vi "DragDropCustomize.vi"(5 "Set Cursor (T)":bool=TRUE, 7 "Function":enum16{"Event", "Cleanup"}(ring), 8 "error in (no error)":errorcluster, 9 "Coords":T2, 10 "CtlRef":refnum<vi>, 11 "Event Type":T3) -> (0 "error out":errorcluster, 1 "InBounds":bool, 2 "CtlRef out":refnum<vi>, 3 "Drag Status":T1, 4 "Bar Cursor ID":refnum<k1>)   [LabVIEW 2021, in "TreeControlLib.lvlib"]
uses:
  TreeControlLib.lvlib
  <vilib>/event_ctls.llb/lveventtype.ctl
  <vilib>/Utility/miscctls.llb/LVPoint32TypeDef.ctl
  ce4e9e53-98d0-488d-9291-147195c1407e.vi
  <vilib>/Utility/cursorutil.llb/Set Cursor (Icon Pict).vi
  <vilib>/Utility/cursorutil.llb/Set Cursor (Cursor ID).vi
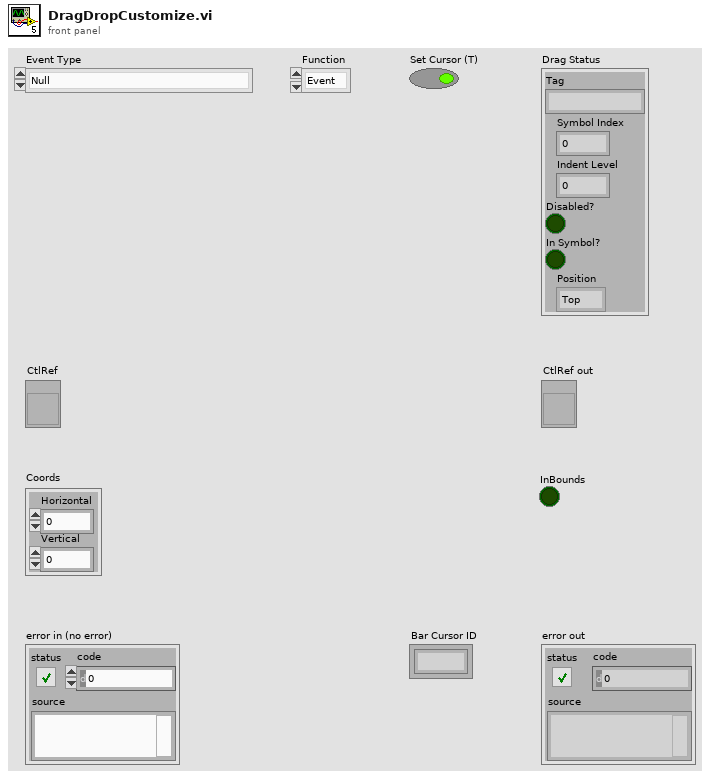
[diagram p1: front panel]
types:
  T1 = cluster{"Tag":string, "Symbol Index":i32, "Indent Level":i32, "Disabled?":bool, "In Symbol?":bool, "Position":enum16{"Top", "Center", "Bottom"}}
  T2 = typedef "LVPoint32TypeDef.ctl" = cluster{"Horizontal":i32, "Vertical":i32}
  T3 = typedef "lveventtype.ctl" = enum32{"Null", "Timeout", "Annotation Menu Selection", "Annotation Menu Selection?", "App Instance Close", "App Instance Close?", "Autoscale Range Change", "Bookmark Info Change", "Cell Edit", "Cell Edit?", "Cursor Grab", "Cursor Grab?", "Cursor Menu Selection", "Cursor Menu Selection?", "Cursor Move", "Cursor Release", "Data Change", "Direction Change", "Display State Change", "Drag Ended", "Drag Enter", "Drag Leave", "Drag Over", "Drag Source Update", "Drag Starting", "Drag Starting?", "Drop", "Exec State Change", "Key Down", "Key Down?", "Key Repeat", "Key Repeat?", "Key Up", "Listbox Double Click", "Menu Activation?", "Menu Selection (App)", "Menu Selection? (App)", "Menu Selection (User)", "Mouse Down", "Mouse Down?", "Mouse Enter", "Mouse Leave", "Mouse Move", "Mouse Up", "Mouse Wheel", "NI Security User Change (App)", "Pane Size", "Panel Close", "Panel Close?", "Panel Resize", "Plot Attribute Change", "Scale Range Change", "Shortcut Menu Activation?", "Shortcut Menu Selection (App)", "Shortcut Menu Selection? (App)", "Shortcut Menu Selection (User)", "Tree Double Click", "Tree Drag", "Tree Drag?", "Tree Drop", "Tree Drop?", "Tree Item Close", "Tree Item Close?", "Tree Item Open", "Tree Item Open?", "User Event", "Value Change"}
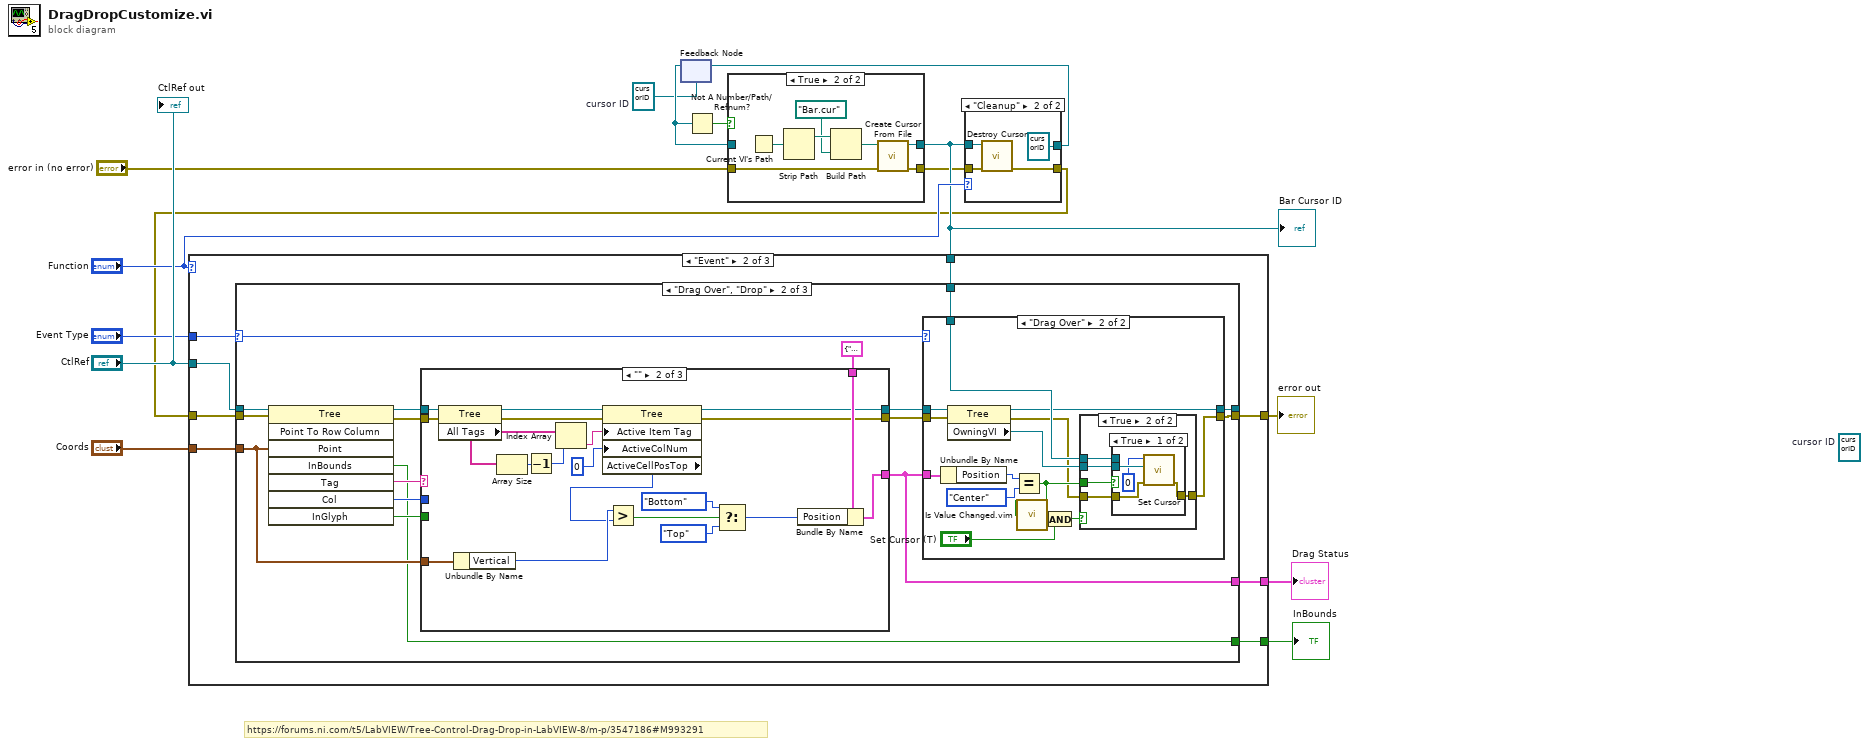
[diagram p0: block diagram]
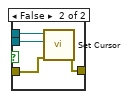
[diagram p6: hidden frame]
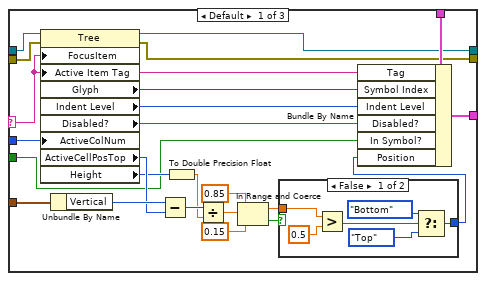
[diagram p7: hidden frame]
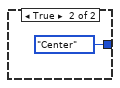
[diagram p8: hidden frame]
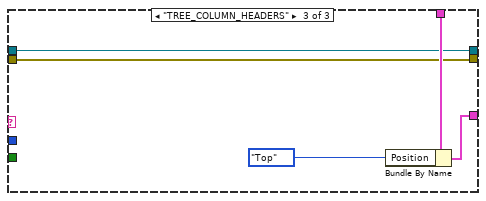
[diagram p9: hidden frame]
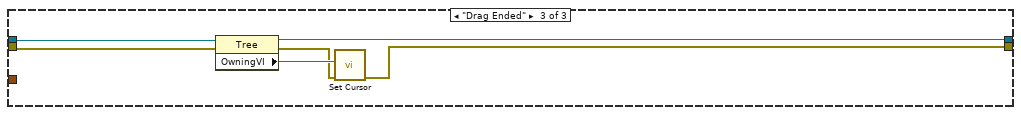
[diagram p10: hidden frame]
diagram:
  w2 = refnum<k1> refnum  # cursor ID
  (unwired) refnum<k1> refnum  # cursor ID
  # "https://forums.ni.com/t5/LabVIEW/Tree-Control-Drag-Drop-in-LabVIEW-8/m-p/3547186#M993291"
  n1 = feedback #1(w2) -> (w14:refnum<k1>)
  n2 = Not A Number/Path/Refnum?(number/path/refnum=w14) -> (NaN/Path/Refnum?=w15:bool)
  n3 = case shown="True" w15 {
    tunnel: w14 -> [w17 _]
    tunnel: [w17 w21] -> w8
    tunnel: "error in (no error)" -> [w16 w20]
    tunnel: [w16 w19] -> w4
    frame False {
    }
    frame True {
      n4 = Current VI's Path() -> (path=w24:path)
      n5 = Strip Path(path=w24) -> (stripped path=w22:path)  [unwired: 1 out]
      n6 = Build Path(base path=w22, name or relative path=path "Bar.cur" ("cursor file")) -> (appended path=w23:path)
      n7 = call <vilib>:"Create Cursor From File.vi"("error in (no error)"=w20, "cursor file"=w23) -> ("error out"=w19:errorcluster, "cursor ID"=w21:refnum<k1>)  [unwired: 8 in]
    }
  }
  "Bar Cursor ID" <- w8
  n8 = case shown="\"Cleanup\"" "Function" {
    tunnel: w8 -> [w26 w30]
    tunnel: [w26 refnum<k1> refnum ("cursor ID")] -> w9
    tunnel: w4 -> [w25 w28]
    tunnel: [w25 w27] -> w3
    frame Default {
    }
    frame "Cleanup" {
      n9 = call <vilib>:"Destroy Cursor.vi"("cursor ID"=w30, "error in (no error)"=w28) -> ("error out"=w27:errorcluster)  [unwired: 8 in]
    }
  }
  n10 = case shown="\"Event\"" "Function" {
    tunnel: "CtlRef" -> [_ w37 _]
    tunnel: "Event Type" -> [_ w38 _]
    tunnel: "Coords" -> [_ w39 _]
    tunnel: w8 -> [_ w36 _]
    tunnel: [_ w35 _] -> w7
    tunnel: [_ w34 _] -> w6
    tunnel: w3 -> [w31 w33 w151]
    tunnel: [w31 w32 w151] -> w1
    frame Default {
    }
    frame "Event" {
      n11 = case shown="\"Drag Over\", \"Drop\"" w38 {
        selector: w38 -> [_ w49 _]
        tunnel: w37 -> [w41 w53 w150]
        tunnel: w39 -> [_ w57 _]
        tunnel: [w41 w48 w148] -> _
        tunnel: w36 -> [_ w50 _]
        tunnel: [_ w47 _] -> w35
        tunnel: [_ w46 _] -> w34
        tunnel: w33 -> [w40 w45 w147]
        tunnel: [w40 w42 w145] -> w32
        frame Default {
        }
        frame "Drag Over", "Drop" {
          n12 = invoke on="Invoke Node" class="Tree" method="Point To Row Column"(reference=w53, error in=w45, "Point"=w57) -> (reference out=w52:refnum<vi>, error out=w44:errorcluster, "InBounds"=w46:bool, "Tag"=w56:string, "Col"=w55:i32, "InGlyph"=w54:bool)  [unwired: 5 in, 2 out]
          n13 = case shown="\"\"" w56 {
            selector: w56 -> [w91 _ _]
            tunnel: w52 -> [w112 w138 w142]
            tunnel: w55 -> [w111 _ _]
            tunnel: w57 -> [w110 w137 _]
            tunnel: w54 -> [w100 _ _]
            tunnel: T1 {"Tag"="", "Symbol Index"=0, "Indent Level"=0, "Disabled?"=FALSE, "In Symbol?"=FALSE, "Position"=enum."Top"} -> [w94 w139 w144]
            tunnel: [w93 w131 w143] -> w47
            tunnel: [w92 w123 w142] -> w51
            tunnel: w44 -> [w90 w130 w140]
            tunnel: [w89 w124 w140] -> w43
            frame Default {
              n14 = property class="Tree"(reference=w112, error in=w90, "FocusItem"=w91, "Active Item Tag"=w91, "ActiveColNum"=w111) -> (reference out=w92:refnum<vi>, error out=w89:errorcluster, "Glyph"=w103:i32, "Indent Level"=w102:i32, "Disabled?"=w101:bool, "ActiveCellPosTop"=w108:i32, "Height"=w106:i32)
              n15 = Unbundle By Name(w110) -> ("Vertical"=w109:i32)
              n16 = Subtract(x=w109, y=w108) -> (x-y=w107:i32)
              n17 = To Double Precision Float(number=w106) -> (double precision float=w105:dbl)
              n18 = Divide(x=w107, y=w105) -> (x/y=w104:dbl)
              n19 = In Range and Coerce(upper limit=0.85, x=w104, lower limit=0.15) -> (coerced(x)=w98:dbl, In Range?=w99:bool)
              n20 = case shown="False" w99 {
                tunnel: w98 -> [w118 _]
                tunnel: [w113 enum16{"Top", "Center", "Bottom"}."Center" ("Position")] -> w95
                frame False {
                  n21 = Greater?(x=w118, y=0.5) -> (0:w116:bool)
                  n22 = Select(t=enum16{"Top", "Center", "Bottom"}."Bottom" ("Position"), s=w116, f=enum16{"Top", "Center", "Bottom"}."Top" ("Position")) -> (s? t:f=w113:enum16{"Top", "Center", "Bottom"})
                }
                frame True {
                }
              }
              n23 = Bundle By Name(cluster=w94, "Tag"=w91, "Symbol Index"=w103, "Indent Level"=w102, "Disabled?"=w101, "In Symbol?"=w100, "Position"=w95) -> (w93:T1)
            }
            frame "" {
              n24 = property class="Tree"(reference=w138, error in=w130) -> (reference out=w126:refnum<vi>, error out=w125:errorcluster, "All Tags"=w129:string[])
              n25 = Unbundle By Name(w137) -> ("Vertical"=w136:i32)
              n26 = Array Size(array=w129) -> (size(s)=w128:i32)
              n27 = Decrement(x=w128) -> (x-1=w127:i32)
              n28 = Index Array(array=w129, index=w127) -> (element=w122:string)
              n29 = property class="Tree"(reference=w126, error in=w125, "Active Item Tag"=w122, "ActiveColNum"=0 ("Active Cell:Active Column Number")) -> (reference out=w123:refnum<vi>, error out=w124:errorcluster, "ActiveCellPosTop"=w120:i32)
              n30 = Greater?(x=w136, y=w120) -> (0:w133:bool)
              n31 = Select(t=enum16{"Top", "Center", "Bottom"}."Bottom" ("Position"), s=w133, f=enum16{"Top", "Center", "Bottom"}."Top" ("Position")) -> (s? t:f=w134:enum16{"Top", "Center", "Bottom"})
              n32 = Bundle By Name(cluster=w139, "Position"=w134) -> (w131:T1)
            }
            frame "TREE_COLUMN_HEADERS" {
              n33 = Bundle By Name(cluster=w144, "Position"=enum16{"Top", "Center", "Bottom"}."Top") -> (w143:T1)
            }
          }
          n34 = case shown="\"Drag Over\"" w49 {
            tunnel: w51 -> [w60 w74]
            tunnel: w47 -> [_ w73]
            tunnel: w50 -> [_ w69]
            tunnel: [w60 w65] -> w48
            tunnel: w43 -> [w59 w66]
            tunnel: [w59 w63] -> w42
            frame Default {
            }
            frame "Drag Over" {
              n35 = Unbundle By Name(w73) -> ("Position"=w72:enum16{"Top", "Center", "Bottom"})
              n36 = property class="Tree"(reference=w74, error in=w66) -> (reference out=w65:refnum<vi>, error out=w64:errorcluster, "OwningVI"=w70:refnum<vi>)
              n37 = Equal?(x=w72, y=enum16{"Top", "Center", "Bottom"}."Center" ("Position")) -> (x = y?=w68:bool)
              n38 = call "Is Value Changed.vim"("value"=w68) -> ("changed or first call?"=w67:bool)
              n39 = And(x=w67, y="Set Cursor (T)") -> (x .and. y?=w62:bool)
              n40 = case shown="True" w62 {
                tunnel: w70 -> [_ w80]
                tunnel: w69 -> [_ w79]
                tunnel: w68 -> [_ w78]
                tunnel: w64 -> [w75 w77]
                tunnel: [w75 w76] -> w63
                frame False {
                }
                frame True {
                  n41 = case shown="True" w78 {
                    tunnel: w80 -> [w84 w88]
                    tunnel: w79 -> [_ w87]
                    tunnel: w77 -> [w82 w86]
                    tunnel: [w81 w85] -> w76
                    frame True {
                      n42 = call-poly <vilib>:"Set Cursor.vi"("error in (no error)"=w82, "VI reference (current VI)"=w84, "icon"=u16 0) -> ("error out"=w81:errorcluster)  [unwired: 7 in, 1 out]
                    }
                    frame False {
                      n43 = call-poly <vilib>:"Set Cursor.vi"("error in (no error)"=w86, "VI reference (current VI)"=w88, "cursor ID"=w87) -> ("error out"=w85:errorcluster)  [unwired: 7 in, 1 out]
                    }
                  }
                }
              }
            }
          }
        }
        frame "Drag Ended" {
          n44 = property class="Tree"(reference=w150, error in=w147) -> (reference out=w148:refnum<vi>, error out=w146:errorcluster, "OwningVI"=w149:refnum<vi>)
          n45 = call-poly <vilib>:"Set Cursor.vi"("error in (no error)"=w146, "VI reference (current VI)"=w149) -> ("error out"=w145:errorcluster)  [unwired: 8 in, 1 out]
        }
      }
    }
    frame "Cleanup" {
      # "上の別枠に処理が書かれている"
    }
  }
  "Drag Status" <- w7
  "InBounds" <- w6
  "error out" <- w1
  n46 = feedback-in #1(w9) -> ()
  "CtlRef out" <- "CtlRef"
